vi "VolumeFilter.vi"(1 "data in":u8[][][](array[numeric]), 2 "window size":i32=3, 3 "threshold":i32) -> (0 "Data Out":u8[][][](array[numeric]))   [LabVIEW 2022 SP3]
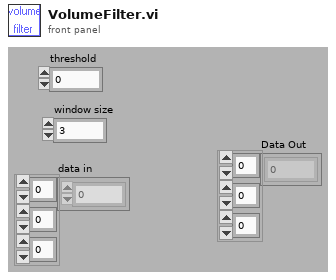
[diagram p1: front panel]
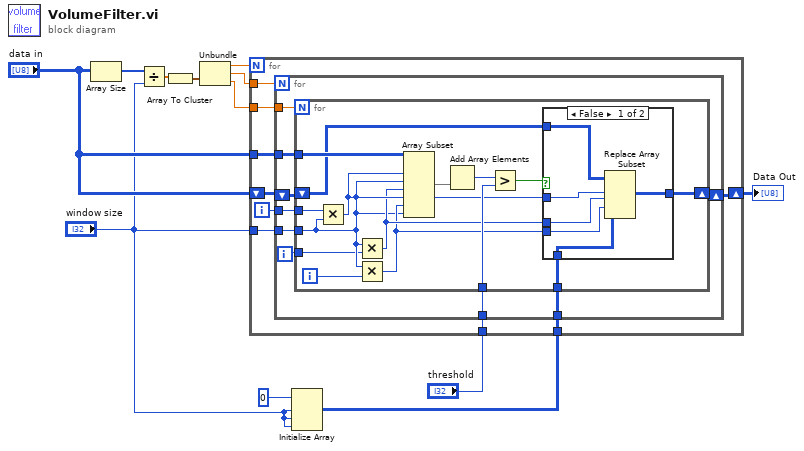
[diagram p0: block diagram]
diagram:
  n1 = Array Size(array="data in") -> (size(s)=w5:i32[])
  n2 = Divide(x=w5, y="window size") -> (x/y=w10:dbl[])
  n3 = Array To Cluster(array=w10) -> (cluster=w11:cluster{"[0]":dbl, "[1]":dbl, "[2]":dbl})
  n4 = Unbundle(w11) -> ("[0]"=w8:dbl, "[1]"=w12:dbl, "[2]"=w7:dbl)
  n5 = Initialize Array(u8 0, "window size", "window size", "window size") -> (w2:u8[][][])
  n6 = for {
    N: w8 -> [_]
    tunnel: "data in" -> [w21]
    tunnel: "threshold" -> [w19]
    shift-right: [w18] -> w9
    shift-left: "data in" -> [w17]
    tunnel: w12 -> [w16]
    tunnel: w7 -> [w15]
    tunnel: w2 -> [w14]
    tunnel: "window size" -> [w13]
    i -> [w20]
    n7 = for {
      N: w16 -> [_]
      tunnel: w21 -> [w30]
      tunnel: w20 -> [w29]
      tunnel: w19 -> [w27]
      shift-right: [w26] -> w18
      shift-left: w17 -> [w25]
      tunnel: w15 -> [w24]
      tunnel: w14 -> [w23]
      tunnel: w13 -> [w22]
      i -> [w28]
      n8 = for {
        N: w24 -> [_]
        tunnel: w30 -> [w37]
        tunnel: w29 -> [w45]
        tunnel: w28 -> [w31]
        tunnel: w27 -> [w44]
        shift-right: [w34] -> w26
        shift-left: w25 -> [w36]
        tunnel: w23 -> [w35]
        tunnel: w22 -> [w32]
        i -> [w33]
        n9 = Multiply(x=w45, y=w32) -> (x*y=w40:i32)
        n10 = Multiply(x=w32, y=w31) -> (x*y=w39:i32)
        n11 = Multiply(x=w32, y=w33) -> (x*y=w38:i32)
        n12 = Array Subset(array=w37, index (dim 0)=w40, length (dim 0)=w32, index (dim 1)=w39, length (dim 1)=w32, index (dim 2)=w38, length (dim 2)=w32) -> (w41:u8[][][])
        n13 = Add Array Elements(numeric array=w41) -> (sum=w43:u8)
        n14 = Greater?(x=w43, y=w44) -> (0:w42:bool)
        n15 = case shown="False" w42 {
          tunnel: w40 -> [w51 _]
          tunnel: w39 -> [w50 _]
          tunnel: w38 -> [w49 _]
          tunnel: w36 -> [w46 w52]
          tunnel: w35 -> [w48 _]
          tunnel: [w47 w52] -> w34
          frame False {
            n16 = Replace Array Subset(array=w46, new element=w48, index (dim 0)=w51, index (dim 1)=w50, index (dim 2)=w49) -> (w47:u8[][][])
          }
          frame True {
          }
        }
      }
    }
  }
  "Data Out" <- w9
